vi "getDuration.vi"(8 "error in (no error)":errorcluster, 11 "StationKeeping in":refnum<class "StationKeeping.lvclass">) -> (0 "error out":errorcluster, 2 "Duration":timestamp, 3 "StationKeeping out":refnum<class "StationKeeping.lvclass">)   [LabVIEW 2013, in "StationKeeping.lvclass"]
uses:
  StationKeeping.lvclass
  StationKeeping.lvclass/StationKeeping.ctl
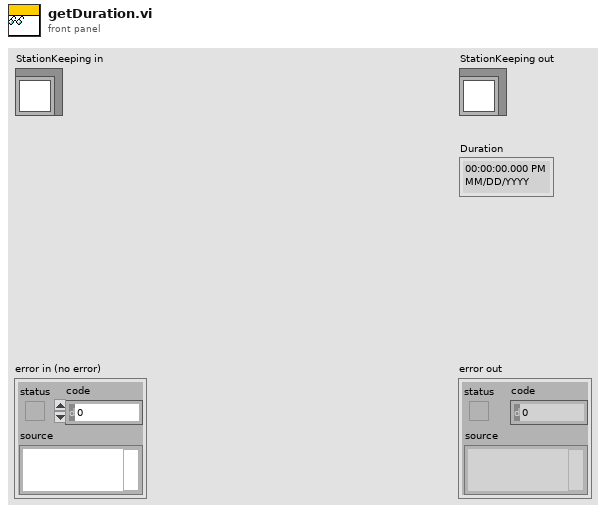
[diagram p1: front panel]
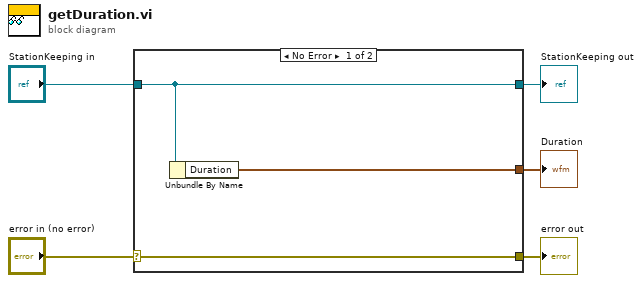
[diagram p0: block diagram]
diagram:
  n1 = case shown="No Error" "error in (no error)" {
    selector: "error in (no error)" -> [w8 w9]
    tunnel: [w8 w9] -> w4
    tunnel: [w7 w10] -> w2
    tunnel: "StationKeeping in" -> [w7 w10]
    tunnel: [w6 _] -> w1
    frame No Error {
      n2 = Unbundle By Name(w7) -> ("Duration"=w6:timestamp)
    }
    frame Error {
    }
  }
  "error out" <- w4
  "StationKeeping out" <- w2
  "Duration" <- w1
